vi "FPGA Accumulate Coil Volts Secondary.vi"(11 "Data Array In":T1=[0, 0]) -> (3 "Data Array Out":T1)   [LabVIEW 2020]
doc: "Author: Scott Hannahs <sth@magnet.fsu.edu>\nCopyright 2018 Florida State University, All rights reserved."
uses:
  SCH Data Controls/SCH Raw Int Data Secondary.ctl
  <vilib>/rvi/eio/common/nirviEmuTemplateMethod_errors.vi
  <vilib>/eio/EIONode/EIONode.xnode
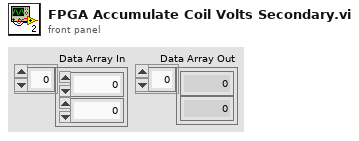
[diagram p1: front panel]
types:
  T1 = typedef "SCH Raw Int Data Secondary.ctl" = i16[]
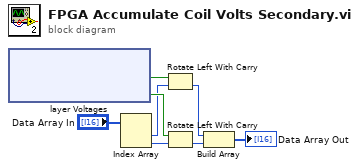
[diagram p0: block diagram]
diagram:
  n1 = xnode "layer Voltages"() -> ("Cold Mass Voltage"=w7:bool, "Cowound Coil"=w8:bool)  [unwired: 2 in, 2 out]
  n2 = Index Array(array="Data Array In") -> (element #1=w5:i16, element #2=w4:i16)  [unwired: 2 in]
  n3 = Rotate Left With Carry(2:w5, 3:w7) -> (0:w3:i16)  [unwired: 1 out]
  n4 = Rotate Left With Carry(2:w4, 3:w8) -> (0:w2:i16)  [unwired: 1 out]
  n5 = Build Array(w3, w2) -> (→"Data Array Out":i16[])
